vi "ReturnToZero.vi"(1 "error in (no error)":errorcluster, 2 "AnalogOut":refnum<k21>[](array[refnum]), 3 "DigitalTasks OUT":refnum<k21>[](array[refnum])) -> (0 "error out":errorcluster)   [LabVIEW 2012]
uses:
  <vilib>/DAQmx/write.llb/DAQmx Write (Digital 1D U32 1Chan NSamp).vi
  <vilib>/DAQmx/write.llb/DAQmx Write (Analog 1D DBL NChan 1Samp).vi
  <vilib>/DAQmx/miscellaneous.llb/DAQmx Fill In Error Info.vi
  <resource>/objmgr/daqmx.rc
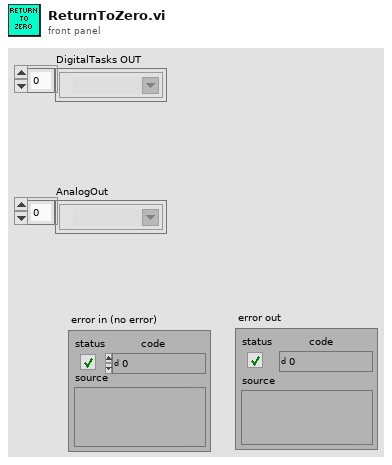
[diagram p1: front panel]
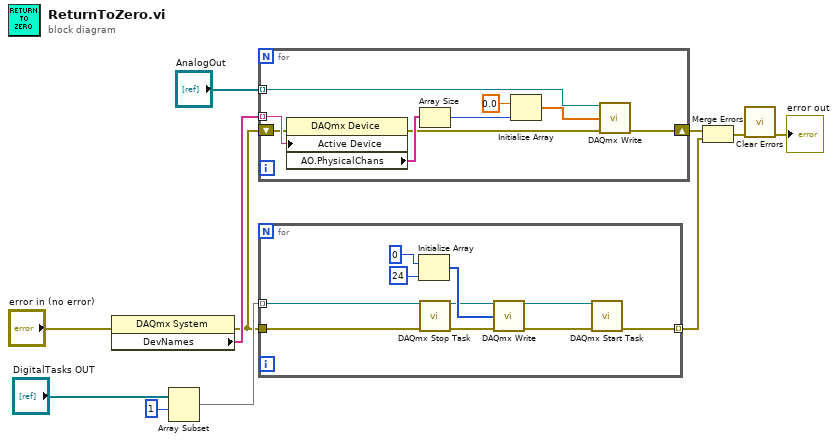
[diagram p0: block diagram]
diagram:
  n1 = property class="DAQmx System"(error in="error in (no error)") -> (error out=w6:errorcluster, "DevNames"=w7:tag[])  [unwired: 1 in, 1 out]
  n2 = Array Subset(array="DigitalTasks OUT", index=1) -> (w9:refnum<k21>[])  [unwired: 1 in]
  n3 = for {
    tunnel: "AnalogOut" -> [w15] mode=indexing
    tunnel: w7 -> [w17] mode=indexing
    shift-right: [w14] -> w11
    shift-left: w6 -> [w12]
    n4 = property class="DAQmx Device"(error in=w12, "Active Device"=w17) -> (error out=w13:errorcluster, "AO.PhysicalChans"=w20:tag[])  [unwired: 1 in, 1 out]
    n5 = Array Size(array=w20) -> (size(s)=w19:i32)
    n6 = Initialize Array(0.0 ("element"), w19) -> (w16:dbl[])
    n7 = call-poly <vilib>:"DAQmx Write.vi"("task/channels in"=w15, "data"=w16, "error in"=w13) -> ("error out"=w14:errorcluster)  [unwired: 10 in, 2 out]
  }
  n8 = for {
    tunnel: w9 -> [w30] mode=indexing
    tunnel: w6 -> [w29]
    tunnel: [w21] -> w5 mode=indexing
    n9 = Initialize Array(u32 0, 24) -> (w26:u32[])
    n10 = call <vilib>:"DAQmx Stop Task.vi"("task/channels in"=w30, "error in"=w29) -> ("task out"=w25:refnum<k21>, "error out"=w24:errorcluster)  [unwired: 12 in]
    n11 = call-poly <vilib>:"DAQmx Write.vi"("task/channels in"=w25, "data"=w26, "error in"=w24) -> ("task out"=w23:refnum<k21>, "error out"=w22:errorcluster)  [unwired: 10 in, 1 out]
    n12 = call <vilib>:"DAQmx Start Task.vi"("task/channels in"=w23, "error in"=w22) -> ("error out"=w21:errorcluster)  [unwired: 12 in, 1 out]
  }
  n13 = Merge Errors(w11, w5) -> (w10:errorcluster)
  n14 = call <vilib>:"Clear Errors.vi"("error in (no error)"=w10) -> ("error out"=→"error out":errorcluster)  [unwired: 6 in]
